vi "guitartuner.vi"() -> ()   [LabVIEW 2025]
uses:
  <vilib>/express/express analysis/Spectral/Block/exnSpectralBlock spectral measurements peak poly.vi
  <vilib>/express/express analysis/Spectral/Block/exnSpectralBlock spectral measurements peak DDT.vi
  <vilib>/express/express analysis/Spectral/XNode/ExpressSpectralMeasurementsBlockNode.xnode
  <vilib>/ptbypt/NI_PtbyPt.lvlib
panel:
  in  "ON/OFF":bool
  out "Frequency Spectrum":dbl[](graph)
  out "Sharp":bool
  out "In Tune":bool
  out "Flat":bool
  out "Target Frequency [Hz]":dbl
  out "Detected frequency [Hz]":dbl
  out "Tuning Status":dbl(knob) scale=-50.0..50.0
  in  "Choose String":T1(ring)
  # "GUITAR TUNER"
  # "How to use"
  # "1. Select String that you want to tune\n\n2.Pluck your \nguitar string\n\n3.Adjust until \"In Tune\""
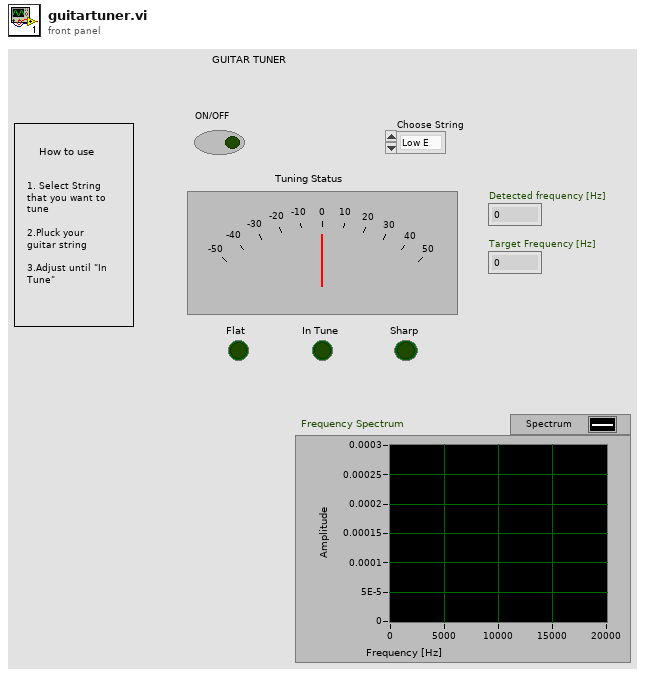
[diagram p1: front panel]
types:
  T1 = enum16{"Low E", "A", "D", "G", "B", "High E", ""}
  T2 = cluster{"averaging mode":u16, "weighting mode":u16, "number of averages":u32}
  T3 = cluster{"dB On (F)":bool, "unwrap phase (F)":bool, "convert to degree (F)":bool}
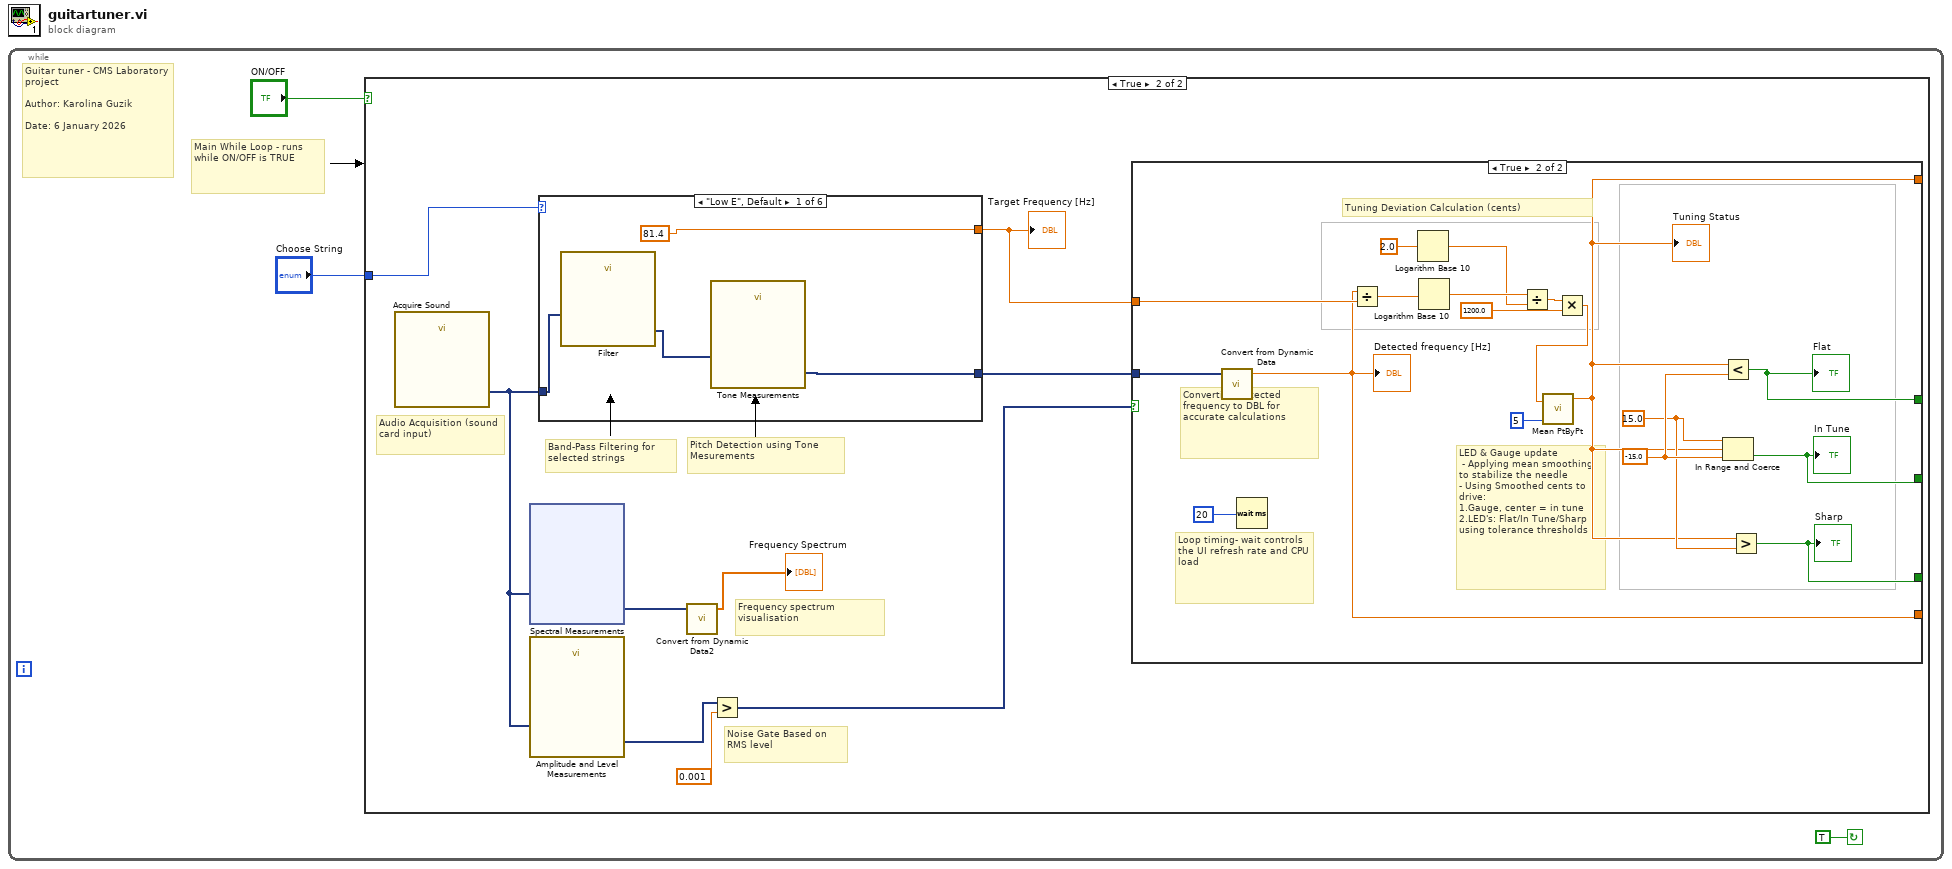
[diagram p0: block diagram]
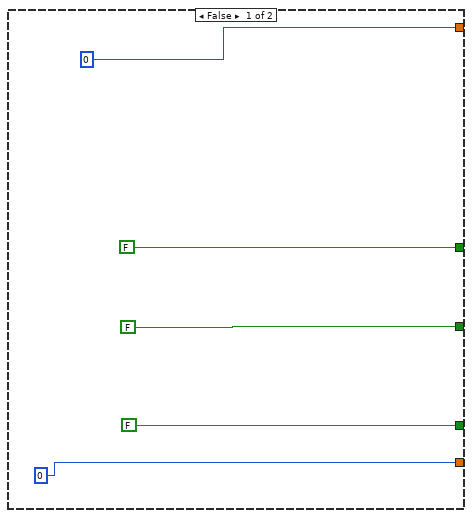
[diagram p3: hidden frame]
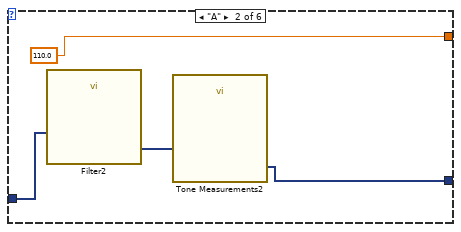
[diagram p4: hidden frame]
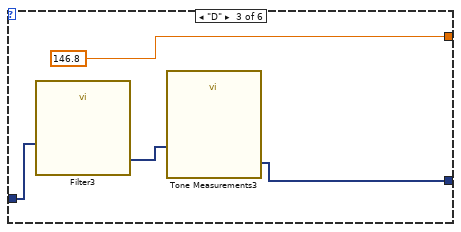
[diagram p5: hidden frame]
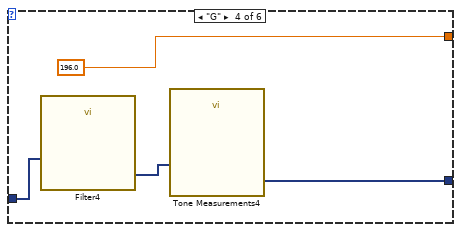
[diagram p6: hidden frame]
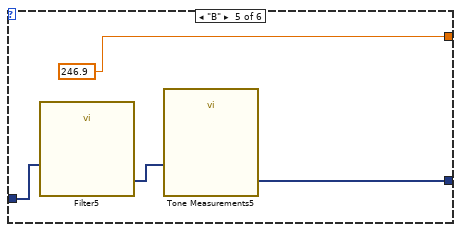
[diagram p7: hidden frame]
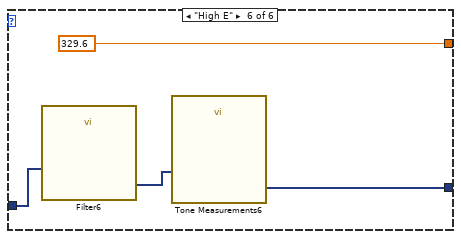
[diagram p8: hidden frame]
diagram:
  n1 = while {
    stop <- TRUE continue-if-true
    # "Guitar tuner - CMS Laboratory project\n\nAuthor: Karolina Guzik\n\nDate: 6 January 2026"
    # "Main While Loop - runs while ON/OFF is TRUE"
    n2 = case shown="True" "ON/OFF" {
      tunnel: "Choose String" -> [_ w12]
      frame False {
      }
      frame True {
        # "Frequency spectrum visualisation"
        # "Noise Gate Based on RMS level"
        # "Pitch Detection using Tone Mesurements"
        # "Band-Pass Filtering for selected strings"
        # "Audio Acquisition (sound card input)"
        n3 = call "Acquire Sound"() -> ("Data"=w6:dynamicdata)  [unwired: 18 in, 1 out]
        n4 = xnode "Spectral Measurements"("Signals"=w6) -> ("FFT - (Peak)"=w11:dynamicdata)  [unwired: 1 in, 2 out]
        n5 = call "Amplitude and Level Measurements"("Signals"=w6) -> ("RMS"=w9:dynamicdata)  [unwired: 13 in, 1 out]
        n6 = case shown="\"Low E\", Default" w12 {
          tunnel: [81.4 110.0 146.8 196.0 246.9 329.6] -> w7
          tunnel: [w46 w51 w55 w59 w63 w66] -> w5
          tunnel: w6 -> [w48 w50 w54 w58 w62 w67]
          frame "Low E", Default {
            n7 = call "Filter"("Signal"=w48) -> ("Filtered Signal"=w47:dynamicdata)  [unwired: 9 in, 1 out]
            n8 = call "Tone Measurements"("Signals"=w47) -> ("Frequency"=w46:dynamicdata)  [unwired: 9 in, 1 out]
          }
          frame "A" {
            n9 = call "Filter2"("Signal"=w50) -> ("Filtered Signal"=w52:dynamicdata)  [unwired: 9 in, 1 out]
            n10 = call "Tone Measurements2"("Signals"=w52) -> ("Frequency"=w51:dynamicdata)  [unwired: 9 in, 1 out]
          }
          frame "D" {
            n11 = call "Filter3"("Signal"=w54) -> ("Filtered Signal"=w56:dynamicdata)  [unwired: 9 in, 1 out]
            n12 = call "Tone Measurements3"("Signals"=w56) -> ("Frequency"=w55:dynamicdata)  [unwired: 9 in, 1 out]
          }
          frame "G" {
            n13 = call "Filter4"("Signal"=w58) -> ("Filtered Signal"=w60:dynamicdata)  [unwired: 9 in, 1 out]
            n14 = call "Tone Measurements4"("Signals"=w60) -> ("Frequency"=w59:dynamicdata)  [unwired: 9 in, 1 out]
          }
          frame "B" {
            n15 = call "Filter5"("Signal"=w62) -> ("Filtered Signal"=w64:dynamicdata)  [unwired: 9 in, 1 out]
            n16 = call "Tone Measurements5"("Signals"=w64) -> ("Frequency"=w63:dynamicdata)  [unwired: 9 in, 1 out]
          }
          frame "High E" {
            n17 = call "Filter6"("Signal"=w67) -> ("Filtered Signal"=w68:dynamicdata)  [unwired: 9 in, 1 out]
            n18 = call "Tone Measurements6"("Signals"=w68) -> ("Frequency"=w66:dynamicdata)  [unwired: 9 in, 1 out]
          }
        }
        "Target Frequency [Hz]" <- w7
        n19 = call "Convert from Dynamic Data2"("Dynamic Data Type"=w11) -> ("Array"=→"Frequency Spectrum":dbl[])  [unwired: 3 in]
        n20 = Greater?(x=w9, y=0.001) -> (0:w4:dynamicdata)
        n21 = case shown="True" w4 {
          tunnel: w7 -> [_ w24]
          tunnel: [0 w22] -> _
          tunnel: [0 w19] -> _
          tunnel: [FALSE w27] -> _
          tunnel: [FALSE w26] -> _
          tunnel: [FALSE w25] -> _
          tunnel: w5 -> [_ w21]
          frame False {
          }
          frame True {
            w28 = 15.0
            w29 = -15.0
            # "Converting detected frequency to DBL for accurate calculations"
            # "Loop timing- wait controls the UI refresh rate and CPU load"
            # "LED & Gauge update \n - Applying mean smoothing to stabilize the needle\n- Using Smoothed cents to drive:\n1.Gauge, center = in tune\n2.LED's: Flat/In Tune/Sharp using tolerance thresholds"
            # "Tuning Deviation Calculation (cents)"
            n22 = call "Convert from Dynamic Data"("Dynamic Data Type"=w21) -> ("Scalar"=w22:dbl)  [unwired: 3 in]
            "Detected frequency [Hz]" <- w22
            n23 = Wait (ms)(milliseconds to wait=20) -> ()  [unwired: 1 out]
            n24 = Divide(x=w22, y=w24) -> (x/y=w34:dbl)
            n25 = Logarithm Base 10(1:2.0) -> (0:w31:dbl)
            n26 = Logarithm Base 10(1:w34) -> (0:w32:dbl)
            n27 = Divide(x=w32, y=w31) -> (x/y=w30:dbl)
            n28 = Multiply(x=w30, y=1200.0) -> (x*y=w20:dbl)
            n29 = call <vilib>:"Mean PtByPt.vi"("x"=w20, "sample length"=5) -> ("mean"=w19:dbl)  [unwired: 2 in, 1 out]
            "Tuning Status" <- w19
            n30 = Less?(x=w19, y=w29) -> (x < y?=w27:bool)
            "Flat" <- w27
            n31 = In Range and Coerce(upper limit=w28, x=w19, lower limit=w29) -> (In Range?=w26:bool)  [unwired: 1 out]
            "In Tune" <- w26
            n32 = Greater?(x=w19, y=w28) -> (0:w25:bool)
            "Sharp" <- w25
          }
        }
      }
    }
  }
